vi "Manual.vi"(6 "Cluster":T11={"VISA resource name"="", "baud rate "=9600}, 7 "vi reference":refnum<vi>, 8 "error in (no error)":errorcluster, 9 "IOList_280":T1, 11 "Manual":T4(tab)) -> (0 "error out":errorcluster, 3 "Out reference":refnum<vi>)   [LabVIEW 2015]
uses:
  Control Button/Exit.ctl
  Control Button/Scanner config.ctl
  Control Button/Save.ctl
  Galobal variable_TI.vi
  <vilib>/addons/database/Connection.llb/DB Tools Open Connec (String).vi
  Project Setup/Globle Variable/GR_Servo.vi
  <vilib>/Instr/_visa.llb/VISA Configure Serial Port (Instr).vi
  <vilib>/addons/database/NI_Database_API.lvlib
panel:
  out "D0List _280":string[](array[string])
  out "LVDT":string
  out "error out 3":errorcluster
  out "Array":string[](array[string])
  out "Byte Lenth":i32
  out "error out 2":errorcluster
  out "Manual DO":bool[](array[boolean])
  in  "Stop":T2
  out "NewVal":T3
  in  "Digital Output":T5
  out "Digital Input":T6
  in  "Home Calling M2":bool
  in  "Home Calling M1":bool
  in  "Stop M2":bool
  in  "Stop M1":bool
  in  "SERVO ON CMD M2":bool
  in  "Speed (mm/s )M2":i32=10
  in  "Travel (mm) M2":i32=5
  in  "SERVO ON CMD M1":bool
  in  "Speed (mm/s) M1":i32=10
  in  "Travel (mm)M1":i32=5
  out "STM1 Done Bit":bool
  out "STM2 Done Bit":bool
  out "Error Message":string
  out "Error Message 2":string
  in  "Sensor Setting Data":T7 {"IL Sensor1_Max AI1" format="%0.02f"; "IL Sensor1_Max AI5" format="%0.02f"; "IL Sensor1_ Min AI1" format="%0.02f"; "IL Sensor1_Min AI4" format="%0.02f"}
  in  "Save":T8
  in  "Analog Input":cluster{"Analog Data":dbl, "Analog Data 2":dbl}
  in  "Sensor Data 2":T9 {"IL Sensor1_AI05" format="%0.02f"; "IL Sensor1_AI04" format="%0.02f"}
  out "Error Status":bool
  in  "Scanner config":T10
  out "Read data":string
  out "Boolean":bool
  # "Instruction for Servo motor Operate\n(1)  Switch  ON -OFF  of Fixture Slide servo Brake ON Cmd (P0.19)  \n      from Digital Output tab.\n(2) Switch  ON -OFF  of Fixture Slide Servo Direction Command (P0.20)\n      from Digital Output tab."
  # "LCD pressing Servo"
  # "Fixture Slide servo"
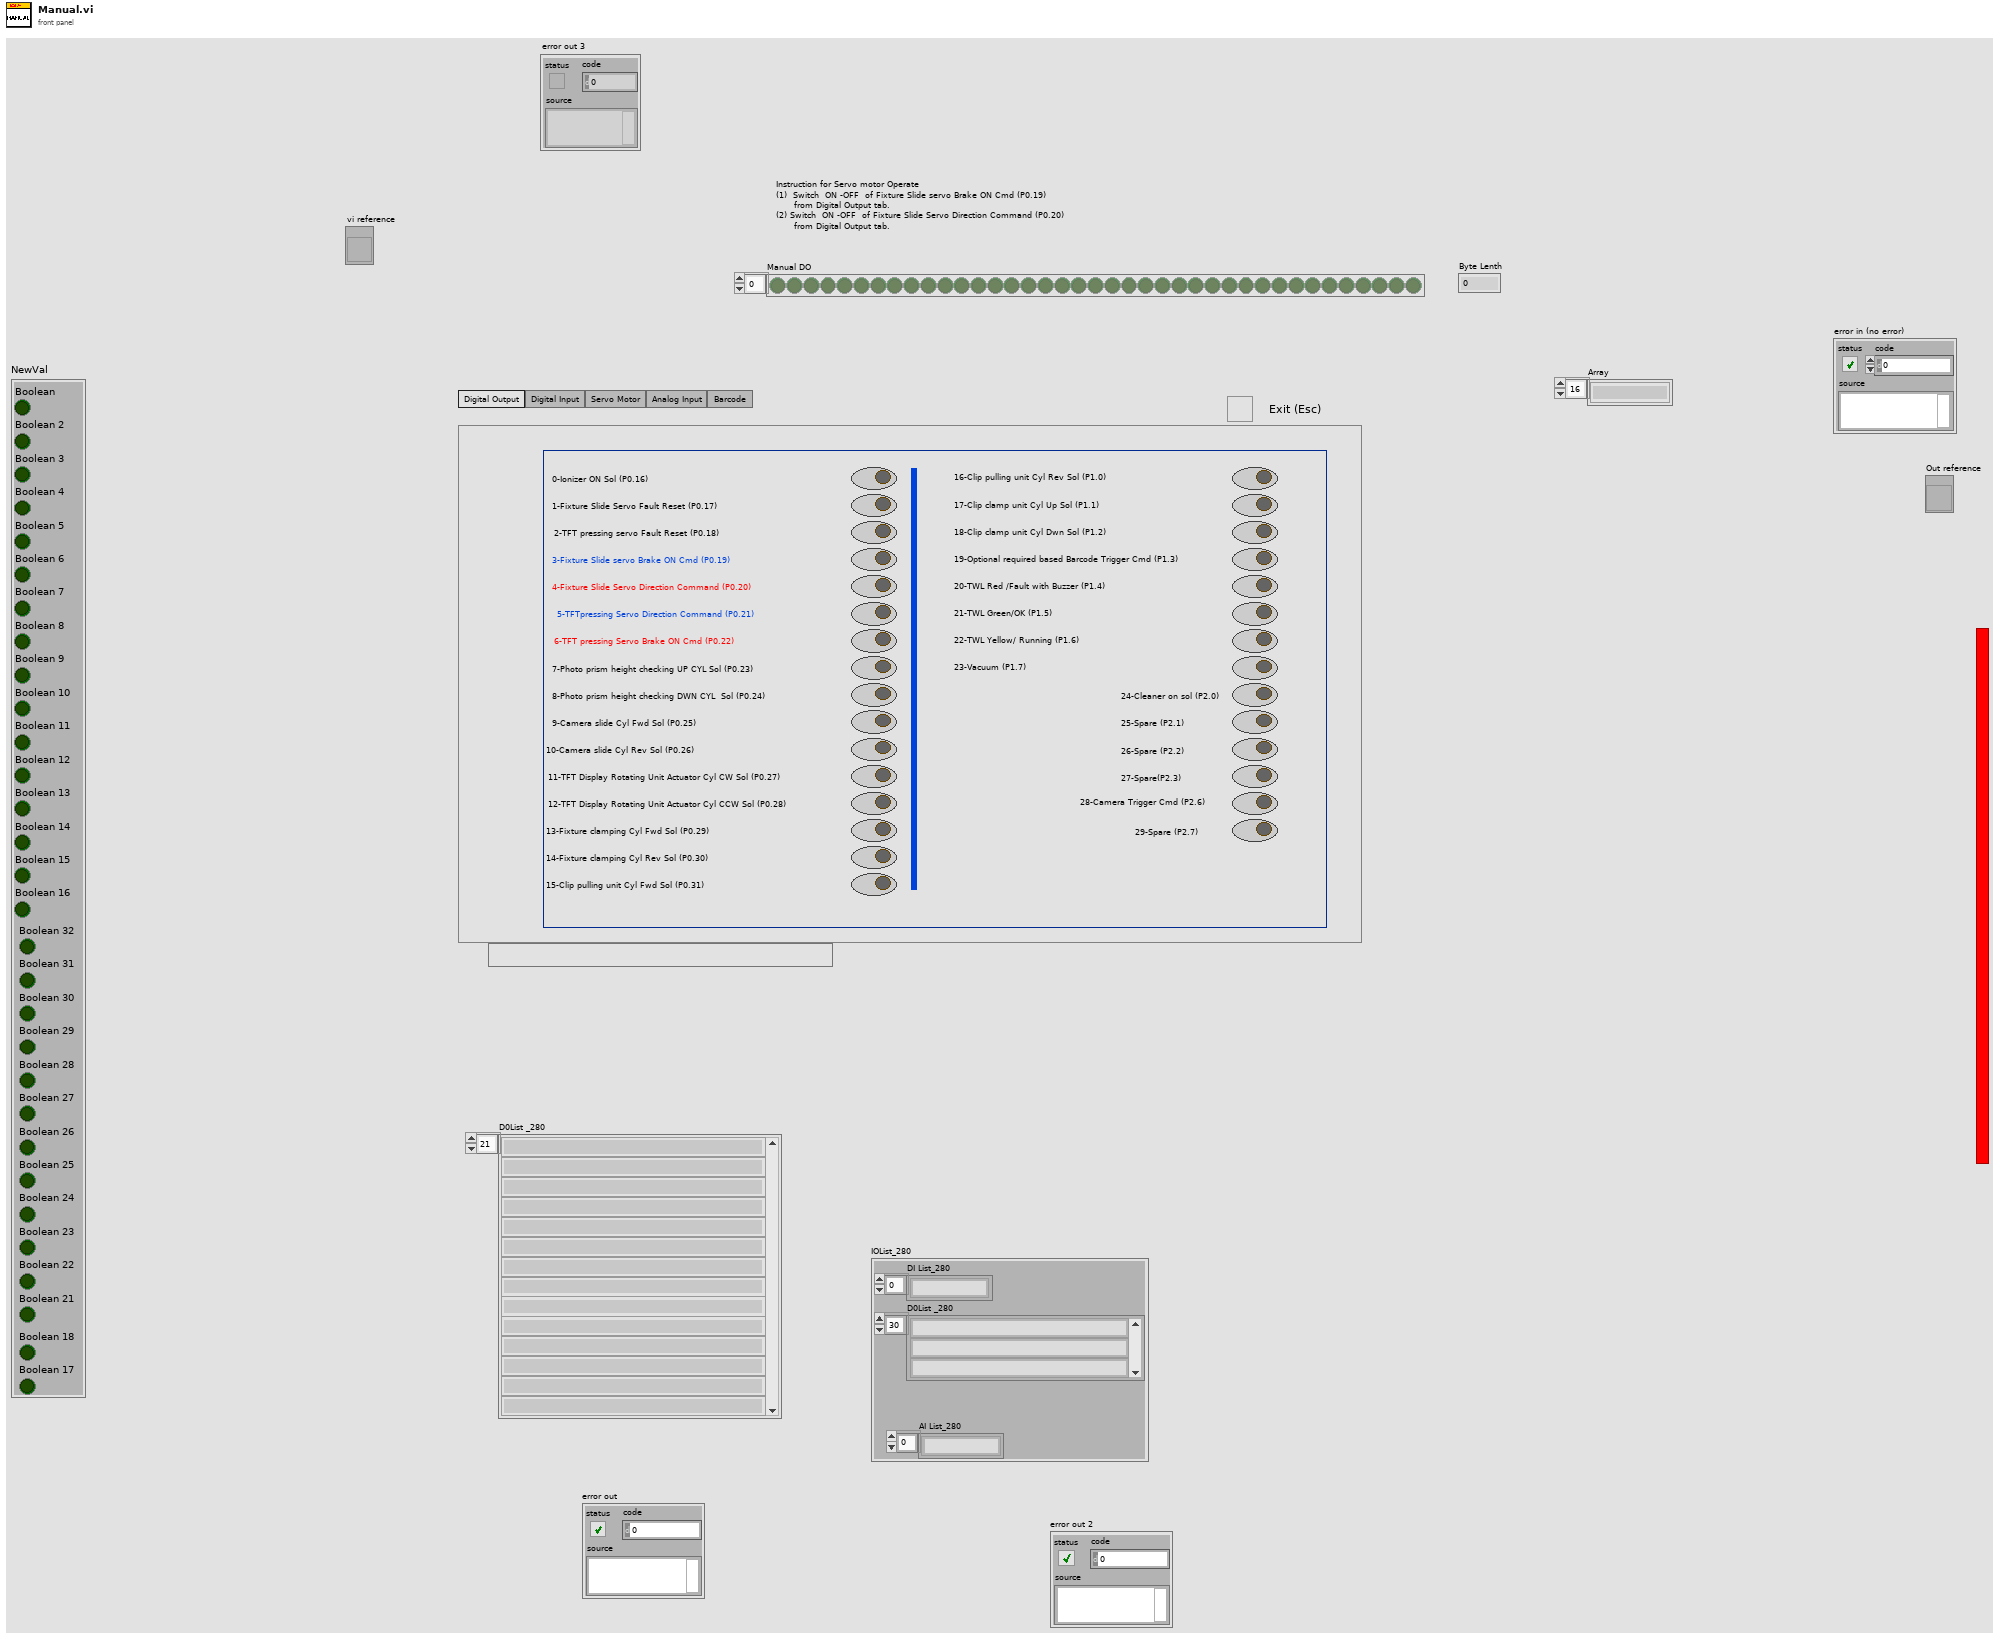
[diagram p1: front panel]
types:
  T1 = cluster{"DI List_280":string[], "D0List _280":string[], "AI List_280":string[]}
  T2 = typedef "Exit.ctl" = bool
  T3 = cluster{"Boolean":bool, "Boolean 2":bool, "Boolean 3":bool, "Boolean 4":bool, "Boolean 5":bool, "Boolean 6":bool, "Boolean 7":bool, "Boolean 8":bool, "Boolean 9":bool, "Boolean 10":bool, "Boolean 11":bool, "Boolean 12":bool, "Boolean 13":bool, "Boolean 14":bool, "Boolean 15":bool, "Boolean 16":bool, "Boolean 17":bool, "Boolean 18":bool, "Boolean 21":bool, "Boolean 22":bool, "Boolean 23":bool, "Boolean 24":bool, "Boolean 25":bool, "Boolean 26":bool, "Boolean 27":bool, "Boolean 28":bool, "Boolean 29":bool, "Boolean 30":bool, "Boolean 31":bool, "Boolean 32":bool}
  T4 = enum32{"Digital Output", "Digital Input", "Servo Motor ", "Analog Input", "Barcode "}
  T5 = cluster{"DO.00":bool, "DO.01":bool, "DO.02":bool, "DO.03":bool, "DO.04":bool, "DO.05":bool, "DO.06":bool, "DO.06":bool, "DO.07":bool, "DO.08":bool, "DO.09":bool, "DO.10":bool, "DO.11":bool, "DO.12":bool, "DO.13":bool, "DO.14":bool, "DO.07 2":bool, "DO.08 2":bool, "DO.09 2":bool, "DO.10 2":bool, "DO.11 2":bool, "DO.12 2":bool, "DO.13 2":bool, "DO.14 2":bool, "DO.00 2":bool, "DO.01 2":bool, "DO.02 2":bool, "DO.03 2":bool, "DO.06 2":bool, "DO.06 3":bool}
  T6 = cluster{"Digital Input":bool, "Digital Input 2":bool, "Digital Input 3":bool, "Digital Input 4":bool, "Digital Input 5":bool, "Digital Input 6":bool, "Digital Input 7":bool, "Digital Input 8":bool, "Digital Input 9":bool, "Digital Input 10":bool, "Digital Input 11":bool, "Digital Input 12":bool, "Digital Input 13":bool, "Digital Input 14":bool, "Digital Input 15":bool, "Digital Input 16":bool, "Digital Input 17":bool, "Digital Input 18":bool, "Digital Input 19":bool, "Digital Input 20":bool, "Digital Input 21":bool, "Digital Input 22":bool, "Digital Input 23":bool, "Digital Input 24":bool, "Digital Input 25":bool, "Digital Input 26":bool, "Digital Input 27":bool, "Digital Input 28":bool, "Digital Input 29":bool, "Digital Input 30":bool, "Digital Input 31":bool, "Digital Input 32":bool, "Digital Input 33":bool, "Digital Input 34":bool, "Digital Input 35":bool, "Digital Input 36":bool, "Digital Input 37":bool, "Digital Input 38":bool, "Digital Input 39":bool, "Digital Input 40":bool, "Digital Input 41":bool, "Digital Input 42":bool, "Digital Input 43":bool, "Digital Input 44":bool}
  T7 = cluster{"IL Sensor1_Max AI5":dbl, "IL Sensor1_Min AI4":dbl, "IL Sensor1_Max AI1":dbl, "IL Sensor1_ Min AI1":dbl}
  T8 = typedef "Save.ctl" = bool
  T9 = cluster{"IL Sensor1_AI04":dbl, "IL Sensor1_AI05":dbl, "IL Sensor1_AI04":bool, "IL Sensor1_AI05":bool}
  T10 = typedef "Scanner config.ctl" = bool
  T11 = cluster{"VISA resource name":refnum<visa-resource-name>, "baud rate ":u32}
  T12 = typedef "NI_Database_API.lvlib/Conn ObjectReference.ctl" = refnum<k1>
  T13 = cluster{"ILSensormax_1":dbl, "ILSensormin_1":dbl, "ILSensormax _2":dbl, "ILSensormin_2":dbl}
  T14 = cluster{"LCD Servo Brack on":refnum<vi>, " LCD  Direction":refnum<vi>, "LCDServo Cmd":refnum<vi>, "LCD Servo Home":refnum<vi>}
  T15 = cluster{" Fixture Brack on":refnum<vi>, " Fixture Direction":refnum<vi>, "Servo Cmd":refnum<vi>, "Servo Home":refnum<vi>}
  T16 = cluster{"ILSensormax_1":dbl, "ILSensormin_1":dbl, "ILSensormax _2":dbl, "ILSensormin_2":dbl, "Key":string}
  T17 = cluster{"Digital input[0]":bool, "Digital input[1]":bool, "Digital input[2]":bool, "Digital input[3]":bool, "Digital input[4]":bool, "Digital input[5]":bool, "Digital input[6]":bool, "Digital input[7]":bool, "Digital input[8]":bool, "Digital input[9]":bool, "Digital input[10]":bool, "Digital input[11]":bool, "Digital input[12]":bool, "Digital input[13]":bool, "Digital input[14]":bool, "Digital input[15]":bool, "Digital input[16]":bool, "Digital input[17]":bool, "Digital input[18]":bool, "Digital input[19]":bool, "Digital input[20]":bool, "Digital input[21]":bool, "Digital input[22]":bool, "Digital input[23]":bool, "Digital input[24]":bool, "Digital input[25]":bool, "Digital input[26]":bool, "Digital input[27]":bool, "Digital input[28]":bool, "Digital input[29]":bool, "Digital input[30]":bool, "Digital input[31]":bool, "Digital input[32]":bool, "Digital input[33]":bool, "Digital input[34]":bool, "Digital input[35]":bool, "Digital input[36]":bool, "Digital input[37]":bool, "Digital input[38]":bool, "Digital input[39]":bool, "Digital input[40]":bool, "Digital input[41]":bool, "Digital input[42]":bool, "Digital input[43]":bool}
  T18 = cluster{"MaxLoad ":dbl, "Min Load":dbl, "MaxDistance(mm)":dbl, "Min Distance(mm)":dbl, "Load Offset":dbl, "Model":string, "Difusser Code":string, "TFT Code ":string, "LVDT Offset":dbl}
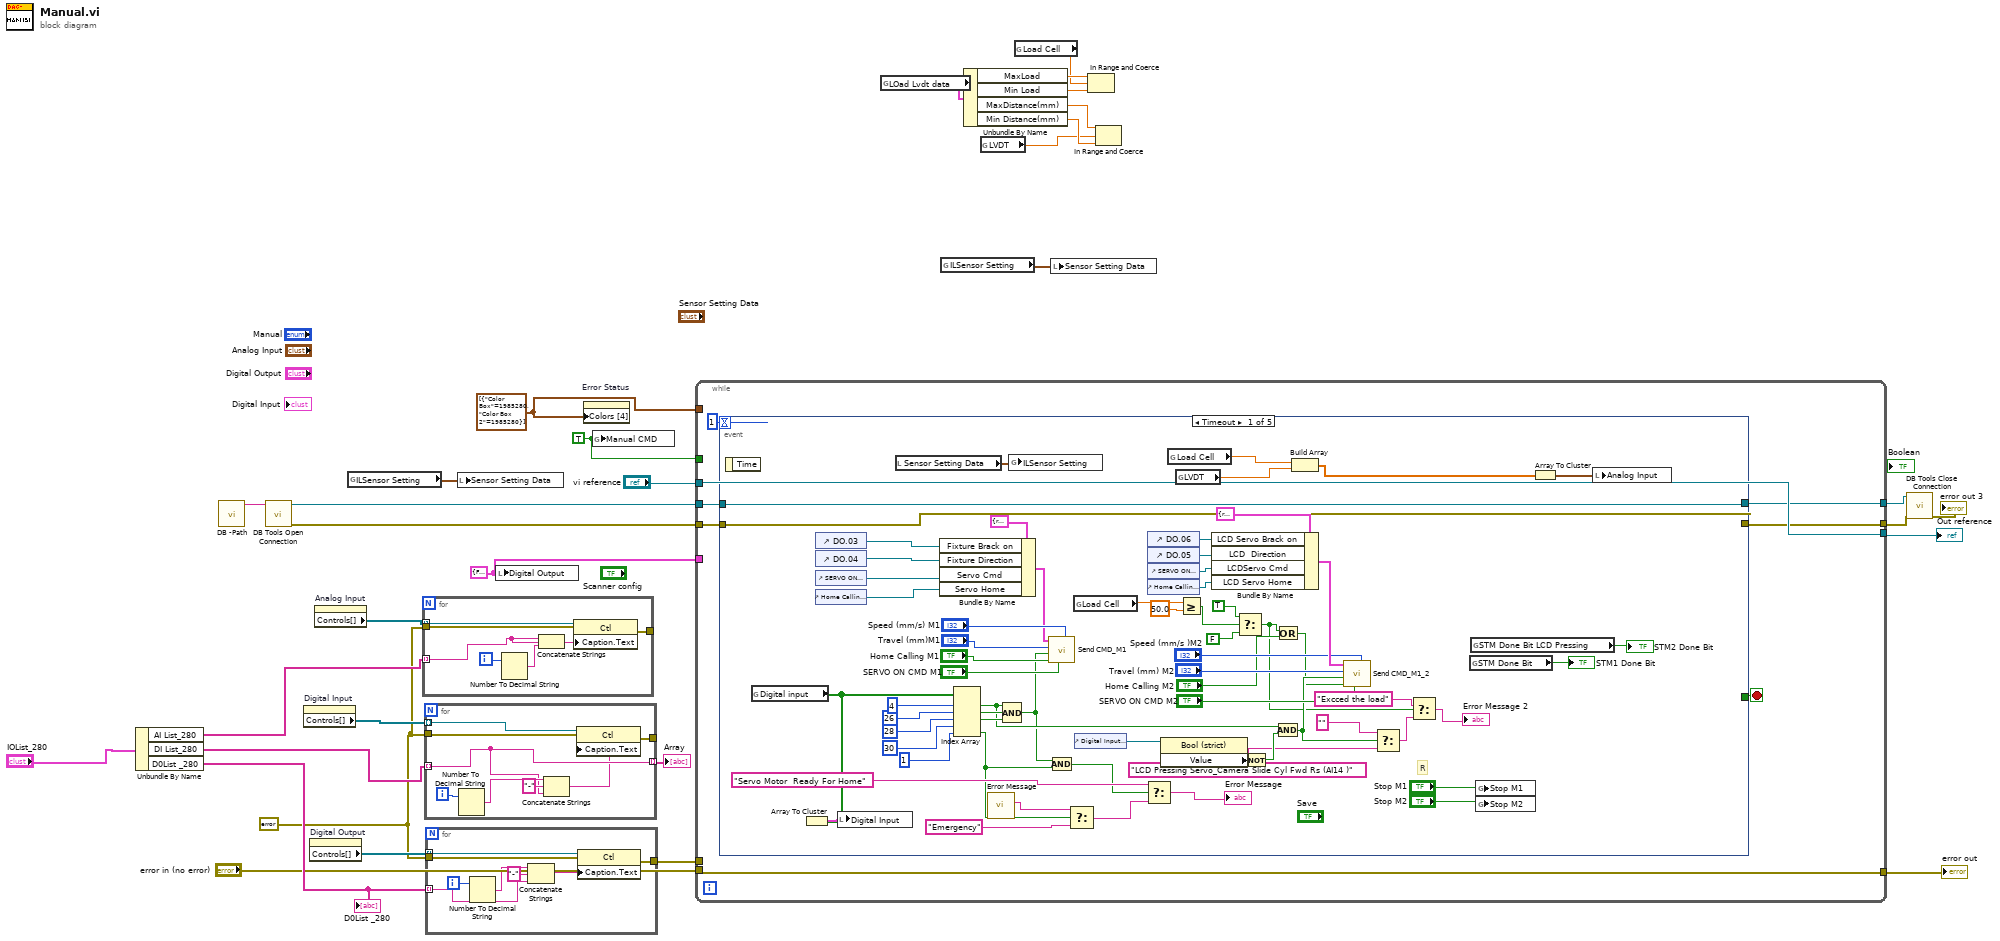
[diagram p0: block diagram]
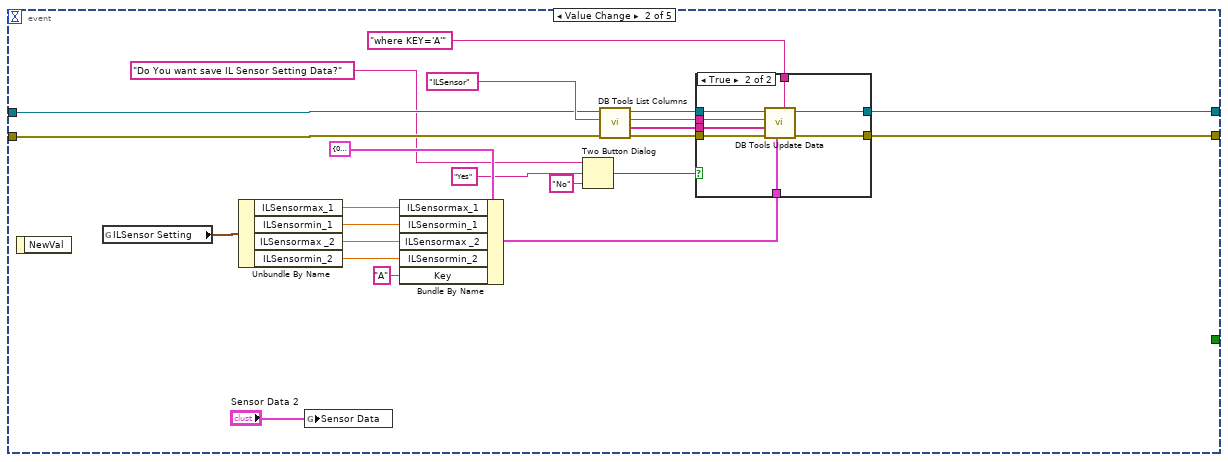
[diagram p2: hidden frame]
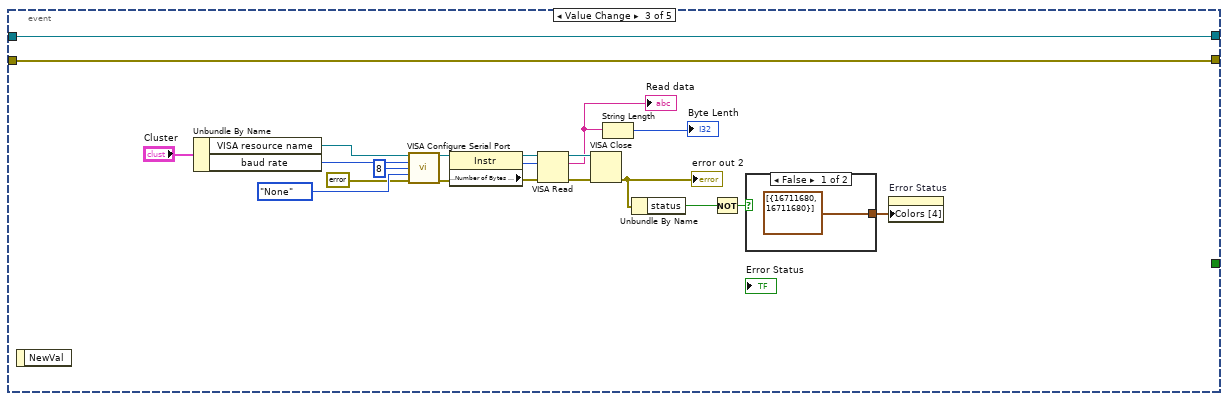
[diagram p4: hidden frame]
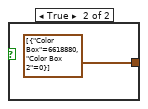
[diagram p5: hidden frame]
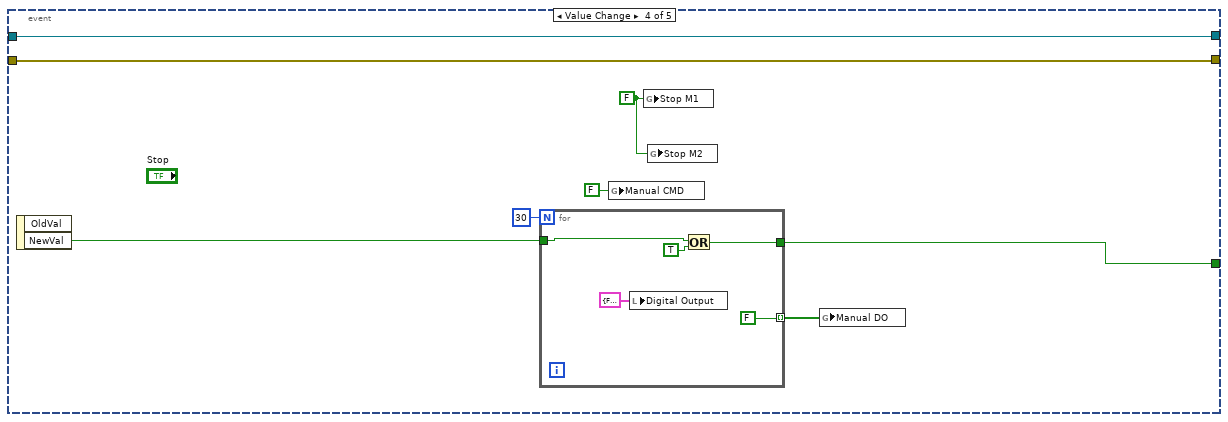
[diagram p6: hidden frame]
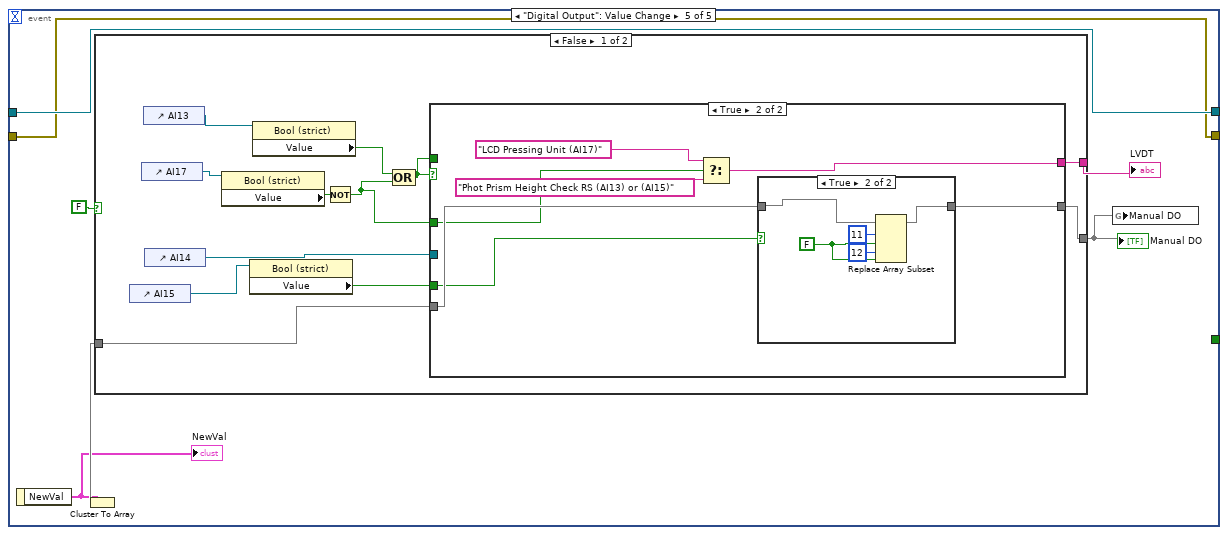
[diagram p7: hidden frame]
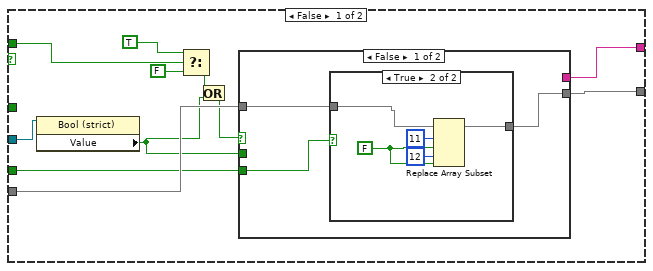
[diagram p8: hidden frame]
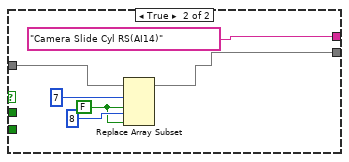
[diagram p10: hidden frame]
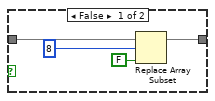
[diagram p11: hidden frame]
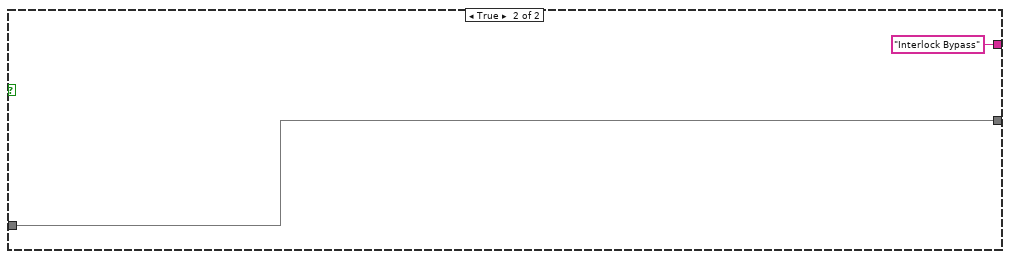
[diagram p12: hidden frame]
diagram:
  w16 = T5 {"DO.00"=FALSE, "DO.01"=FALSE, "DO.02"=FALSE, "DO.03"=FALSE, "DO.04"=FALSE, "DO.05"=FALSE, "DO.06"=FALSE, "DO.06"=FALSE, "DO.07"=FALSE, "DO.08"=FALSE, "DO.09"=FALSE, "DO.10"=FALSE, "DO.11"=FALSE, "DO.12"=FALSE, "DO.13"=FALSE, "DO.14"=FALSE, "DO.07 2"=FALSE, "DO.08 2"=FALSE, "DO.09 2"=FALSE, "DO.10 2"=FALSE, "DO.11 2"=FALSE, "DO.12 2"=FALSE, "DO.13 2"=FALSE, "DO.14 2"=FALSE, "DO.00 2"=FALSE, "DO.01 2"=FALSE, "DO.02 2"=FALSE, "DO.03 2"=FALSE, "DO.06 2"=FALSE, "DO.06 3"=FALSE} ("Digital Output")
  w19 = errorcluster {"status"=FALSE, "code"=0, "source"=""} ("error in (no error)")
  w22 = cluster{"Color Box":u32, "Color Box 2":u32}[] [{"Color Box"=1985280, "Color Box 2"=1985280}] ("Colors [4]")
  w28 = TRUE ("Manual CMD")
  n1 = Unbundle By Name("IOList_280") -> ("AI List_280"=w23:string[], "DI List_280"=w25:string[], "D0List _280"=w27:string[])
  "D0List _280" <- w27
  n2 = call "DB -Path.vi"() -> ("String"=w15:string)  [unwired: 11 in]
  n3 = call-poly <vilib>:"DB Tools Open Connection.vi"("connection information"=w15) -> ("error out"=w13:errorcluster, "connection reference"=w14:T12)  [unwired: 7 in]
  n4 = property on="Digital Input" class="Clust (strict)"() -> ("Controls[]"=w26:refnum<vi>[])  [unwired: 2 in, 2 out]
  n5 = property on="Digital Output" class="Clust (strict)"() -> ("Controls[]"=w31:refnum<vi>[])  [unwired: 2 in, 2 out]
  n6 = property on="Analog Input" class="Clust (strict)"() -> ("Controls[]"=w24:refnum<vi>[])  [unwired: 2 in, 2 out]
  n7 = global read "Galobal variable_TI.vi" "ILSensor Setting"() -> (w10:T13)
  n8 = for {
    tunnel: w24 -> [w38] mode=indexing
    tunnel: [w36] -> _
    tunnel: w19 -> [w34]
    tunnel: w23 -> [w33] mode=indexing
    i -> [w37]
    n9 = Number To Decimal String(number=w37) -> (decimal integer string=w35:string)  [unwired: 1 in]
    n10 = Concatenate Strings(w33, w35) -> ()  [unwired: 1 out]
    n11 = property class="Ctl"(reference=w38, error in=w34, "Caption.Text"=w33) -> (error out=w36:errorcluster)  [unwired: 1 out]
  }
  n12 = for {
    tunnel: w26 -> [w46] mode=indexing
    tunnel: [w44] -> _
    tunnel: w19 -> [w42]
    tunnel: w25 -> [w40] mode=indexing
    tunnel: [w40] -> w20 mode=indexing
    i -> [w45]
    n13 = Number To Decimal String(number=w45) -> (decimal integer string=w43:string)  [unwired: 1 in]
    n14 = Concatenate Strings(w43, "-" ("string"), w40) -> (w39:string)
    n15 = property class="Ctl"(reference=w46, error in=w42, "Caption.Text"=w39) -> (error out=w44:errorcluster)  [unwired: 1 out]
  }
  "Array" <- w20
  n16 = for {
    tunnel: w31 -> [w54] mode=indexing
    tunnel: [w52] -> w32
    tunnel: w19 -> [w50]
    tunnel: w27 -> [w48] mode=indexing
    i -> [w53]
    n17 = Number To Decimal String(number=w53) -> (decimal integer string=w51:string)  [unwired: 1 in]
    n18 = Concatenate Strings(w51, "-" ("string"), w48) -> (w47:string)
    n19 = property class="Ctl"(reference=w54, error in=w50, "Caption.Text"=w47) -> (error out=w52:errorcluster)  [unwired: 1 out]
  }
  n20 = local write "Sensor Setting Data"(w10) -> ()
  n21 = local write "Digital Output"(w16) -> ()
  n22 = property on="Error Status" class="Bool (strict)"("Colors [4]"=w22) -> ()  [unwired: 2 in, 2 out]
  n23 = global write "Galobal variable_TI.vi" "Manual CMD"(w28) -> ()
  n24 = while {
    tunnel: w32 -> [_]
    tunnel: [w60] -> w30
    tunnel: "vi reference" -> [w61]
    tunnel: [w61] -> w29
    tunnel: w28 -> [_]
    tunnel: w22 -> [_]
    tunnel: "error in (no error)" -> [w60]
    tunnel: w16 -> [_]
    tunnel: w14 -> [w58]
    tunnel: w13 -> [w57]
    tunnel: [w56] -> w12
    tunnel: [w55] -> w11
    stop <- w59 stop-if-true
    n25 = event shown="[0] Timeout" {
      selector: _ -> [_ _ _ _ _]
      dyn-events: _ -> [_ _ _ _ _]
      timeout: 1 -> [_ _ _ _ _]
      tunnel: [_ _ _ w185 _] -> w59
      tunnel: w58 -> [w93 w137 w161 w184 w197]
      tunnel: w57 -> [w92 w135 w160 w183 w196]
      tunnel: [w93 w149 w161 w184 w197] -> w56
      tunnel: [w92 w148 w160 w183 w196] -> w55
      event Timeout {
        # "R"
        n26 = event-data() -> ()  [unwired: 1 in, 1 out]
        n27 = global read "Galobal variable_TI.vi" "Digital input"() -> (w104:bool[])
        n28 = Array To Cluster(array=w104) -> (cluster=w127:T17)
        n29 = control-ref of="DO.03"() -> (w118:refnum<vi>)
        n30 = control-ref of="DO.04"() -> (w117:refnum<vi>)
        n31 = control-ref of="SERVO ON CMD M1"() -> (w115:refnum<vi>)
        n32 = control-ref of="Home Calling M1"() -> (w116:refnum<vi>)
        n33 = local write "Digital Input"(w127) -> ()
        n34 = local read "Sensor Setting Data"() -> (w91:T7)
        n35 = Bundle By Name(cluster=T15 {" Fixture Brack on"=refnum, " Fixture Direction"=refnum, "Servo Cmd"=refnum, "Servo Home"=refnum} ("Slide Servo"), "Fixture Brack on"=w118, "Fixture Direction"=w117, "Servo Cmd"=w115, "Servo Home"=w116) -> (w114:T15)
        n36 = Index Array(array=w104, index #1=4 ("index"), index #2=26 ("index"), index #3=28 ("index"), index #4=30 ("index"), index #5=1 ("index")) -> (element #1=w97:bool, element #2=w100:bool, element #3=w99:bool, element #5=w85:bool)  [unwired: 1 out]
        n37 = call "Error Message.vi"() -> ("Error"=w88:string)  [unwired: 11 in]
        n38 = Compound Arithmetic op=AND(w97, w100, w99) -> (w86:bool)
        n39 = global write "Galobal variable_TI.vi" "ILSensor Setting"(w91) -> ()
        n40 = call "Send CMD_M1.vi"("Speed (mm/s) M1"="Speed (mm/s) M1", "SERVO ON CMD M1"="SERVO ON CMD M1", "Home Calling M1"="Home Calling M1", "Pokayoka"=w86, "Travel (mm)M1"="Travel (mm)M1", "Slide Servo"=w114) -> ()  [unwired: 6 in]
        n41 = Compound Arithmetic op=AND(w86, w85) -> (w84:bool)
        n42 = Select(t=w88, s=w85, f="Emergency") -> (s? t:f=w87:string)
        n43 = global read "Galobal variable_TI.vi" "Load Cell"() -> (w73:dbl)
        n44 = control-ref of="Digital Input 29"() -> (w83:refnum<vi>)
        n45 = Select(t="Servo Motor  Ready For Home", s=w84, f=w87) -> (s? t:f=→"Error Message":string)
        n46 = control-ref of="DO.06"() -> (w110:refnum<vi>)
        n47 = control-ref of="DO.05"() -> (w111:refnum<vi>)
        n48 = control-ref of="SERVO ON CMD M2"() -> (w108:refnum<vi>)
        n49 = control-ref of="Home Calling M2"() -> (w109:refnum<vi>)
        n50 = property class="Bool (strict)"(reference=w83) -> ("Value"=w82:bool)  [unwired: 1 in, 2 out]
        n51 = global read "Galobal variable_TI.vi" "Load Cell"() -> (w77:dbl)
        n52 = global read "Galobal variable_TI.vi" "LVDT"() -> (w76:dbl)
        n53 = Greater Or Equal?(x=w73, y=50.0) -> (x >= y?=w71:bool)
        n54 = Bundle By Name(cluster=T14 {"LCD Servo Brack on"=refnum, " LCD  Direction"=refnum, "LCDServo Cmd"=refnum, "LCD Servo Home"=refnum} ("LCD Pressing Servo"), "LCD Servo Brack on"=w110, "LCD  Direction"=w111, "LCDServo Cmd"=w108, "LCD Servo Home"=w109) -> (w112:T14)
        n55 = Select(t=TRUE, s=w71, f=FALSE) -> (s? t:f=w66:bool)
        n56 = Not(x=w82) -> (.not. x?=w81:bool)
        n57 = Or(x=w66, y="Home Calling M2") -> (x .or. y?=w67:bool)
        n58 = Compound Arithmetic op=AND(w97, w81) -> (w80:bool)
        n59 = Build Array(w77, w76) -> (w74:dbl[])
        n60 = call "Send CMD_M1_2.vi"("Speed (mm/s) M1"="Speed (mm/s )M2", "SERVO ON CMD M1"="SERVO ON CMD M2", "Home Calling M1"=w67, "Pokayoka"=w80, "Travel (mm)M1"="Travel (mm) M2", "LCD Pressing Servo"=w112) -> ()  [unwired: 6 in]
        n61 = Select(t="", s=w80, f="LCD Pressing Servo_Camera Slide Cyl Fwd Rs (AI14 )") -> (s? t:f=w64:string)
        n62 = Select(t="Excced the load", s=w66, f=w64) -> (s? t:f=→"Error Message 2":string)
        n63 = global read "Galobal variable_TI.vi" "STM Done Bit"() -> (→"STM1 Done Bit":bool)
        n64 = global read "GR_Servo.vi" "STM Done Bit LCD Pressing"() -> (→"STM2 Done Bit":bool)
        n65 = global write "Galobal variable_TI.vi" "Stop M1"("Stop M1") -> ()
        n66 = global write "Galobal variable_TI.vi" "Stop M2"("Stop M2") -> ()
        n67 = Array To Cluster(array=w74) -> (cluster=w75:cluster{"[0]":dbl, "[1]":dbl})
        n68 = local write "Analog Input"(w75) -> ()
      }
      event Value Change {
        w138 = "ILSensor" ("table")
        n69 = event-data() -> ()  [unwired: 1 in, 1 out]
        n70 = global read "Galobal variable_TI.vi" "ILSensor Setting"() -> (w128:T13)
        n71 = Unbundle By Name(w128) -> ("ILSensormax_1"=w145:dbl, "ILSensormin_1"=w144:dbl, "ILSensormax _2"=w143:dbl, "ILSensormin_2"=w142:dbl)
        n72 = global write "Galobal variable_TI.vi" "Sensor Data"("Sensor Data 2") -> ()
        n73 = Bundle By Name(cluster=T16 {"ILSensormax_1"=0.0, "ILSensormin_1"=0.0, "ILSensormax _2"=0.0, "ILSensormin_2"=0.0, "Key"="A"} ("ILSensor Setting"), "ILSensormax_1"=w145, "ILSensormin_1"=w144, "ILSensormax _2"=w143, "ILSensormin_2"=w142, "Key"="A") -> (w139:T16)
        n74 = Two Button Dialog(message="Do You want save IL Sensor Setting Data?", 1:"No" ("F button name (\"Cancel\")"), 2:"Yes" ("T button name (\"OK\")")) -> (T button?=w132:bool)
        n75 = call <vilib>:"DB Tools List Columns.vi"("error in (no error)"=w135, "table"=w138, "connection reference"=w137) -> ("error out"=w134:errorcluster, "columns"=w133:string[], "connection reference out"=w136:T12)  [unwired: 1 in, 1 out]
        n76 = case shown="True" w132 {
          tunnel: [w151 w159] -> w149
          tunnel: [w150 w158] -> w148
          tunnel: "where KEY='A'" ("condition") -> [_ w157]
          tunnel: w139 -> [_ w156]
          tunnel: w138 -> [_ w155]
          tunnel: w136 -> [w151 w154]
          tunnel: w134 -> [w150 w153]
          tunnel: w133 -> [_ w152]
          frame False {
          }
          frame True {
            n77 = call <vilib>:"DB Tools Update Data.vi"("condition"=w157, "data"=w156, "error in (no error)"=w153, "columns"=w152, "table"=w155, "connection reference"=w154) -> ("error out"=w158:errorcluster, "connection reference out"=w159:T12)  [unwired: 4 in]
          }
        }
      }
      event Value Change {
        n78 = event-data() -> ()  [unwired: 1 in, 1 out]
        n79 = Unbundle By Name("Cluster") -> ("VISA resource name"=w180:refnum<visa-resource-name>, "baud rate"=w179:u32)
        n80 = call-poly "VISA Configure Serial Port"("VISA resource name"=w180, "baud rate (9600)"=w179, "data bits (8)"=u16 8, "parity (0:none)"=enum16{"None", "Odd", "Even", "Mark", "Space"}."None", "error in (no error)"=errorcluster {"status"=FALSE, "code"=0, "source"=""} ("error in (no error) 2")) -> ("VISA resource name out"=w178:refnum<visa-resource-name>, "error out"=w176:errorcluster)  [unwired: 9 in]
        n81 = property class="Instr"(reference=w178, error in=w176) -> (reference out=w177:refnum<visa-resource-name>, error out=w175:errorcluster, "Serial Settings:Number of Bytes at Serial Port"=w174:u32)
        n82 = VISA Read(VISA resource name=w177, byte count=w174, error in (no error)=w175) -> (VISA resource name out=w172:refnum<visa-resource-name>, read buffer=w170:string, error out=w171:errorcluster)  [unwired: 1 out]
        "Read data" <- w170
        n83 = VISA Close(VISA resource name=w172, error in (no error)=w171) -> (error out=w168:errorcluster)
        "error out 2" <- w168
        n84 = String Length(string=w170) -> (length=→"Byte Lenth":i32)
        n85 = Unbundle By Name(w168) -> ("status"=w167:bool)
        n86 = Not(x=w167) -> (.not. x?=w165:bool)
        n87 = case shown="False" w165 {
          tunnel: [cluster{"Color Box":u32, "Color Box 2":u32}[] [{"Color Box"=16711680, "Color Box 2"=16711680}] ("Colors [4]") cluster{"Color Box":u32, "Color Box 2":u32}[] [{"Color Box"=6618880, "Color Box 2"=0}] ("Colors [4]")] -> w166
          frame False {
          }
          frame True {
          }
        }
        n88 = property on="Error Status" class="Bool (strict)"("Colors [4]"=w166) -> ()  [unwired: 2 in, 2 out]
      }
      event Value Change {
        w189 = FALSE ("Stop M1")
        n89 = event-data() -> ("NewVal"=w186:T2)  [unwired: 1 in, 1 out]
        n90 = for {
          N: 30 -> [_]
          tunnel: [FALSE] -> w188 mode=indexing
          tunnel: w186 -> [w193]
          tunnel: [w192] -> w185
          n91 = local write "Digital Output"(T5 {"DO.00"=FALSE, "DO.01"=FALSE, "DO.02"=FALSE, "DO.03"=FALSE, "DO.04"=FALSE, "DO.05"=FALSE, "DO.06"=FALSE, "DO.06"=FALSE, "DO.07"=FALSE, "DO.08"=FALSE, "DO.09"=FALSE, "DO.10"=FALSE, "DO.11"=FALSE, "DO.12"=FALSE, "DO.13"=FALSE, "DO.14"=FALSE, "DO.07 2"=FALSE, "DO.08 2"=FALSE, "DO.09 2"=FALSE, "DO.10 2"=FALSE, "DO.11 2"=FALSE, "DO.12 2"=FALSE, "DO.13 2"=FALSE, "DO.14 2"=FALSE, "DO.00 2"=FALSE, "DO.01 2"=FALSE, "DO.02 2"=FALSE, "DO.03 2"=FALSE, "DO.06 2"=FALSE, "DO.06 3"=FALSE} ("Digital Output")) -> ()
          n92 = Or(x=w193, y=TRUE) -> (x .or. y?=w192:T2)
        }
        n93 = global write "Galobal variable_TI.vi" "Manual CMD"(FALSE ("Manual CMD")) -> ()
        n94 = global write "Galobal variable_TI.vi" "Stop M1"(w189) -> ()
        n95 = global write "Galobal variable_TI.vi" "Stop M2"(w189) -> ()
        n96 = global write "Galobal variable_TI.vi" "Manual DO"(w188) -> ()
      }
      event "Digital Output": Value Change {
        n97 = event-data() -> ("NewVal"=w198:T5)  [unwired: 1 in]
        "NewVal" <- w198
        n98 = Cluster To Array(cluster=w198) -> (array=w199:bool[])
        n99 = case shown="False" FALSE ("By Pass") {
          tunnel: [w213 w258] -> w202
          tunnel: [w211 "Interlock Bypass"] -> w201
          tunnel: w199 -> [w204 w258]
          frame False {
            n100 = control-ref of="AI15"() -> (w205:refnum<vi>)
            n101 = control-ref of="AI17"() -> (w208:refnum<vi>)
            n102 = control-ref of="AI13"() -> (w212:refnum<vi>)
            n103 = control-ref of="AI14"() -> (w214:refnum<vi>)
            n104 = property class="Bool (strict)"(reference=w208) -> ("Value"=w209:bool)  [unwired: 1 in, 2 out]
            n105 = property class="Bool (strict)"(reference=w205) -> ("Value"=w203:bool)  [unwired: 1 in, 2 out]
            n106 = property class="Bool (strict)"(reference=w212) -> ("Value"=w210:bool)  [unwired: 1 in, 2 out]
            n107 = Not(x=w209) -> (.not. x?=w207:bool)
            n108 = Compound Arithmetic op=OR(w210, w207) -> (w206:bool)
            n109 = case shown="True" w206 {
              tunnel: w204 -> [w225 w247]
              tunnel: w214 -> [w224 _]
              tunnel: [w223 w246] -> w213
              tunnel: [w222 w242] -> w211
              tunnel: w207 -> [_ w245]
              tunnel: w206 -> [w221 _]
              tunnel: w203 -> [w215 w241]
              frame False {
                n110 = property class="Bool (strict)"(reference=w224) -> ("Value"=w217:bool)  [unwired: 1 in, 2 out]
                n111 = Select(t=TRUE, s=w221, f=FALSE) -> (s? t:f=w218:bool)
                n112 = Or(x=w218, y=w217) -> (x .or. y?=w216:bool)
                n113 = case shown="False" w216 {
                  tunnel: w225 -> [w227 w238]
                  tunnel: [w226 w237] -> w223
                  tunnel: w217 -> [_ _]
                  tunnel: [_ "Camera Slide Cyl RS(AI14)"] -> w222
                  tunnel: w215 -> [w228 _]
                  frame False {
                    n114 = case shown="True" w228 {
                      tunnel: w227 -> [w229 w232]
                      tunnel: [w229 w231] -> w226
                      frame False {
                      }
                      frame True {
                        w230 = FALSE ("new element/subarray")
                        n115 = Replace Array Subset(array=w232, new element #1=w230, index #1=11 ("index"), new element #2=w230, index #2=12 ("index")) -> (w231:bool[])
                      }
                    }
                  }
                  frame True {
                    w235 = FALSE ("new element/subarray")
                    n116 = Replace Array Subset(array=w238, new element #1=w235, index #1=7 ("index"), new element #2=w235, index #2=8 ("index")) -> (w237:bool[])
                  }
                }
              }
              frame True {
                n117 = Select(t="LCD Pressing Unit (AI17)", s=w245, f="Phot Prism Height Check RS (AI13) or (AI15)") -> (s? t:f=w242:string)
                n118 = case shown="True" w241 {
                  tunnel: w247 -> [w251 w254]
                  tunnel: [w250 w253] -> w246
                  frame False {
                    n119 = Replace Array Subset(array=w251, new element=FALSE ("new element/subarray"), index=8) -> (w250:bool[])
                  }
                  frame True {
                    w252 = FALSE ("new element/subarray")
                    n120 = Replace Array Subset(array=w254, new element #1=w252, index #1=11 ("index"), new element #2=w252, index #2=12 ("index")) -> (w253:bool[])
                  }
                }
              }
            }
          }
          frame True {
          }
        }
        "Manual DO" <- w202
        "LVDT" <- w201
        n121 = global write "Galobal variable_TI.vi" "Manual DO"(w202) -> ()
      }
    }
  }
  "error out" <- w30
  "Out reference" <- w29
  n122 = global read "Galobal variable_TI.vi" "LOad Lvdt data"() -> (w7:T18)
  n123 = global read "Galobal variable_TI.vi" "ILSensor Setting"() -> (w9:T13)
  n124 = Unbundle By Name(w7) -> ("MaxLoad"=w6:dbl, "Min Load"=w5:dbl, "MaxDistance(mm)"=w3:dbl, "Min Distance(mm)"=w2:dbl)
  n125 = global read "Galobal variable_TI.vi" "LVDT"() -> (w1:dbl)
  n126 = global read "Galobal variable_TI.vi" "Load Cell"() -> (w4:dbl)
  n127 = local write "Sensor Setting Data"(w9) -> ()
  n128 = In Range and Coerce(upper limit=w6, x=w4, lower limit=w5) -> ()  [unwired: 2 out]
  n129 = In Range and Coerce(upper limit=w3, x=w1, lower limit=w2) -> ()  [unwired: 2 out]
  n130 = call <vilib>:"DB Tools Close Connection.vi"("error in (no error)"=w11, "connection reference"=w12) -> ("error out"=→"error out 3":errorcluster)  [unwired: 5 in]
